vi "Get Target.vi"(8 "error in (no error)":errorcluster, 11 "Instrument.1820 in":refnum<class "Instrument.Oxford1820.lvclass">) -> (0 "error out":errorcluster, 1 "Target Field Rate (T/min)":dbl, 2 "Target Field (T)":dbl, 3 "Instrument.1820 in":refnum<class "Instrument.Oxford1820.lvclass">)   [LabVIEW 2019, in "Instrument.Oxford1820.lvclass"]
uses:
  Instrument.Oxford1820.lvclass
  Typedefs/Instrument.Oxford1820.Commands-enum.ctl
  2a741720-dfc8-4982-b19f-246f04608042.vi
  <userlib>/LevyLab/Levylab Instruments/Instrument Types/Cryostat/Typedefs/Magnet Mode--Enum.ctl
  <userlib>/LevyLab/Levylab Instruments/Instrument Types/Cryostat/Instrument.Cryostat.lvclass
  <userlib>/LevyLab/Levylab Instruments/Instrument Types/Cryostat/Typedefs/Magnet Axis--Enum.ctl
  <userlib>/LevyLab/Levylab Instruments/Instrument Types/Cryostat/Typedefs/Set Magnet--cluster.ctl
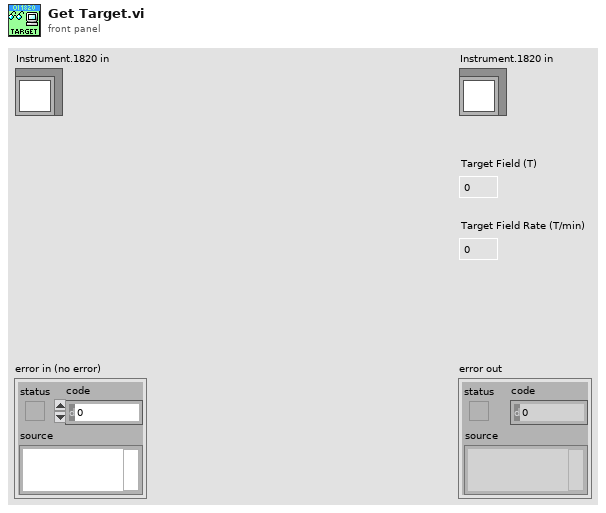
[diagram p1: front panel]
types:
  T1 = typedef "Instrument.Cryostat.lvclass/Set Magnet--cluster.ctl" = cluster{"Field (T)":dbl, "Rate (T/min)":dbl, "Axis":T2, "Mode":T3}
  T2 = typedef "Instrument.Cryostat.lvclass/Magnet Axis--Enum.ctl" = enum16{"Z", "X", "Y"}
  T3 = typedef "Instrument.Cryostat.lvclass/Magnet Mode--Enum.ctl" = enum16{"Persistent", "Driven"}
  T4 = typedef "Instrument.Oxford1820.lvclass/Instrument.Oxford1820.Commands-enum.ctl" = enum16{"setAction", "setTarget", "setSwitchHeat", "setLambda", "setFillMode", "setNeedleValve", "setMagnetField", "getStatus", "getTarget", "getSwitchHeat", "getPSUField", "newcommand", "getMagnetField"}
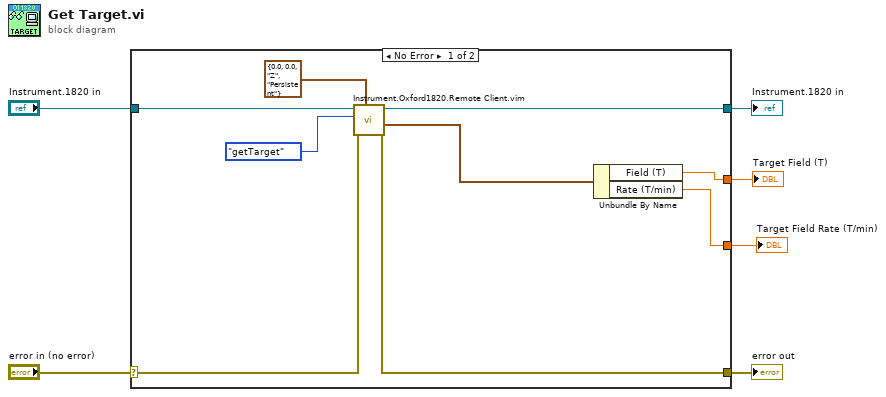
[diagram p0: block diagram]
diagram:
  n1 = case shown="No Error" "error in (no error)" {
    selector: "error in (no error)" -> [w14 w17]
    tunnel: [w9 w17] -> w5
    tunnel: [w10 w16] -> w3
    tunnel: "Instrument.1820 in" -> [w11 w16]
    tunnel: [w13 _] -> w2
    tunnel: [w12 _] -> w1
    frame No Error {
      n2 = call "Instrument.Oxford1820.Remote Client.vim"("Data Out type"=T1 {"Field (T)"=0.0, "Rate (T/min)"=0.0, "Axis"=enum."Z", "Mode"=enum."Persistent"} ("Set Magnet Field"), "error in (no error)"=w14, "Commands"=Instrument.Oxford1820.Commands-enum."getTarget", "Instrument.1820 in"=w11) -> ("error out"=w9:errorcluster, "Data out"=w8:T1, "Instrument.1820 out"=w10:refnum<class "Instrument.Oxford1820.lvclass">)  [unwired: 5 in]
      n3 = Unbundle By Name(w8) -> ("Field (T)"=w13:dbl, "Rate (T/min)"=w12:dbl)
    }
    frame Error {
    }
  }
  "error out" <- w5
  "Instrument.1820 in" <- w3
  "Target Field (T)" <- w2
  "Target Field Rate (T/min)" <- w1
